vi "Read (Euler Angles).vi"(0 "VISA resource name":refnum<visa-resource-name>, 11 "error in (no error)":errorcluster) -> (2 "Checksum Pass":bool, 3 "Timer":u32, 4 "VISA resource name out":refnum<visa-resource-name>, 6 "Roll":sgl, 8 "Pitch":sgl, 10 "Yaw":sgl, 15 "error out":errorcluster)   [LabVIEW 2012, in "MicroStrain 3DM-GXx.lvlib"]
doc: "Read the Euler Angles (Roll, Pitch, Yaw)."
uses:
  <instrlib>/MicroStrain 3DM-GXx/MicroStrain 3DM-GXx.lvlib
  <instrlib>/MicroStrain 3DM-GXx/Public/Data/Parse Message VIs/Parse (Euler Angles).vi
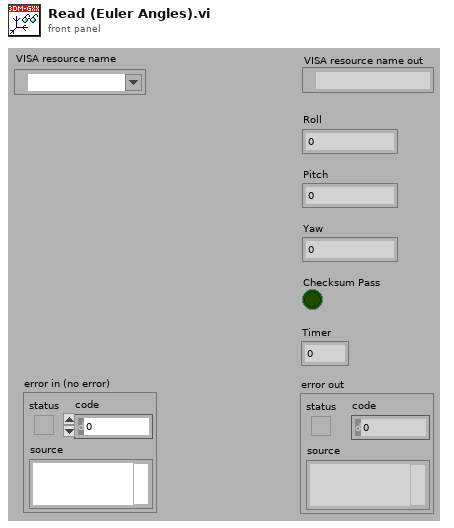
[diagram p1: front panel]
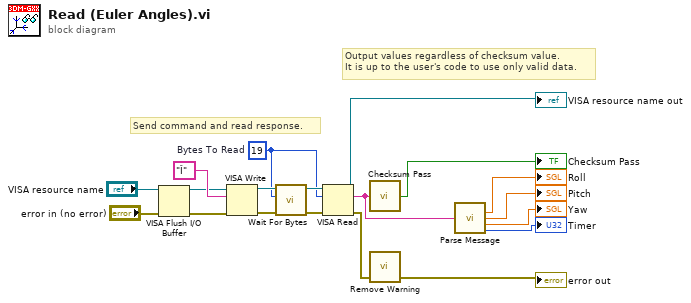
[diagram p0: block diagram]
diagram:
  w14 = u32 19  # Bytes To Read
  # "Output values regardless of checksum value.\nIt is up to the user's code to use only valid data."
  # "Send command and read response."
  n1 = VISA Flush I/O Buffer(VISA resource name="VISA resource name", error in (no error)="error in (no error)") -> (VISA resource name out=w2:refnum<visa-resource-name>, error out=w1:errorcluster)  [unwired: 1 in]
  n2 = VISA Write(VISA resource name=w2, write buffer="Î", error in (no error)=w1) -> (VISA resource name out=w18:refnum<visa-resource-name>, error out=w17:errorcluster)  [unwired: 1 out]
  n3 = call <instrlib>:"Wait For Bytes.vi"("error in (no error)"=w17, "Bytes To Read (0)"=w14, "VISA resource name"=w18) -> ("error out"=w16:errorcluster, "VISA resource name out"=w15:refnum<visa-resource-name>)  [unwired: 7 in]
  n4 = VISA Read(VISA resource name=w15, byte count=w14, error in (no error)=w16) -> (VISA resource name out=→"VISA resource name out":refnum<visa-resource-name>, read buffer=w13:string, error out=w10:errorcluster)  [unwired: 1 out]
  n5 = call <instrlib>:"Checksum Pass.vi"("Message In"=w13) -> ("Checksum Pass"=→"Checksum Pass":bool)  [unwired: 4 in]
  n6 = call <instrlib>:"Remove Warning.vi"("error in (no error)"=w10) -> ("error out"=→"error out":errorcluster)  [unwired: 3 in, 1 out]
  n7 = call-poly <instrlib>:"Parse Message.vi"("Message In"=w13) -> ("Roll"=→"Roll":sgl, "Pitch"=→"Pitch":sgl, "Yaw"=→"Yaw":sgl, "Timer"=→"Timer":u32)  [unwired: 11 in]
